vi "Next Step.vi"(8 "error in (no error)":errorcluster, 11 "Scanner in":refnum<class "Scanner.lvclass">) -> (0 "error out":errorcluster, 1 "Current Step":u32, 2 "Current Position":dbl, 3 "Scanner out":refnum<class "Scanner.lvclass">)   [LabVIEW 2023, in "Scanner.lvclass"]
doc: "(Dynamic) Move to the next preconfigured step of this Scanner, and return the current position (actual, not intended) of this Scanner. Increment the step counter by one."
uses:
  Scanner.lvclass
  Scanner.lvclass/Scanner.ctl
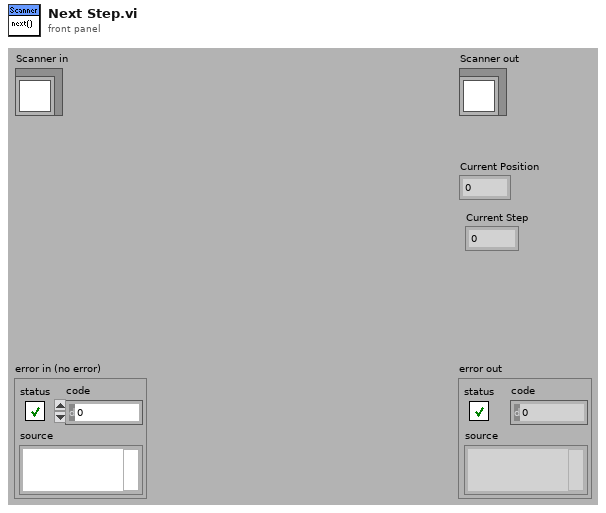
[diagram p1: front panel]
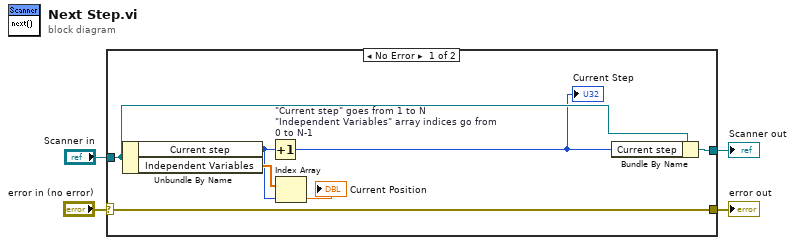
[diagram p0: block diagram]
diagram:
  n1 = case shown="No Error" "error in (no error)" {
    selector: "error in (no error)" -> [w11 w12]
    tunnel: [w11 w12] -> w2
    tunnel: [w10 w13] -> w1
    tunnel: "Scanner in" -> [w9 w13]
    frame No Error {
      n2 = Unbundle By Name(w9) -> ("Current step"=w6:u32, "Independent Variables"=w8:dbl[])
      n3 = Increment "\"Current step\" goes from 1 to N\n\"Independent Variables\" array indices go from 0 to N-1"(x=w6) -> (x+1=w7:u32)
      "Current Step" <- w7
      n4 = Index Array(array=w8, index=w6) -> (element=→"Current Position":dbl)
      n5 = Bundle By Name(cluster=w9, "Current step"=w7) -> (w10:refnum<class "Scanner.lvclass">)
    }
    frame Error {
    }
  }
  "error out" <- w2
  "Scanner out" <- w1
